vi "Stop Process.vi"(8 "error in (no error)":errorcluster, 11 "DLP2 in":refnum<class "DLP2.lvclass">) -> (0 "error out":errorcluster, 3 "DLP2 out":refnum<class "DLP2.lvclass">)   [LabVIEW 2022 SP3, in "DLP2.lvclass"]
doc: "Developed by Kevin Thompson\nkevin@thompsonengineering.net\n\nCopyright 2018\nThompson Engineering, LLC"
uses:
  DLP2.lvclass
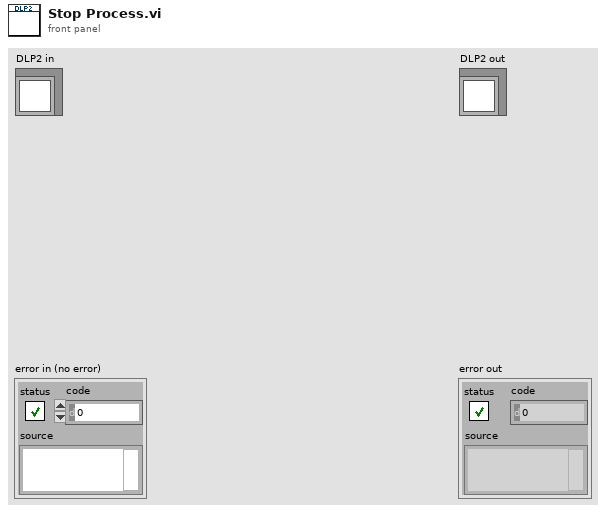
[diagram p1: front panel]
types:
  T1 = typedef "DLP2.lvclass/Public Events--cluster.ctl" = cluster{"Temp01.AsyncCmd Event":refnum<user-event>, "Temp01.AsyncMsg Event":refnum<user-event>, "stop process":refnum<user-event>, "API Incoming Event":refnum<user-event>, "API Executed Event":refnum<user-event>, "API Return Event":refnum<user-event>}
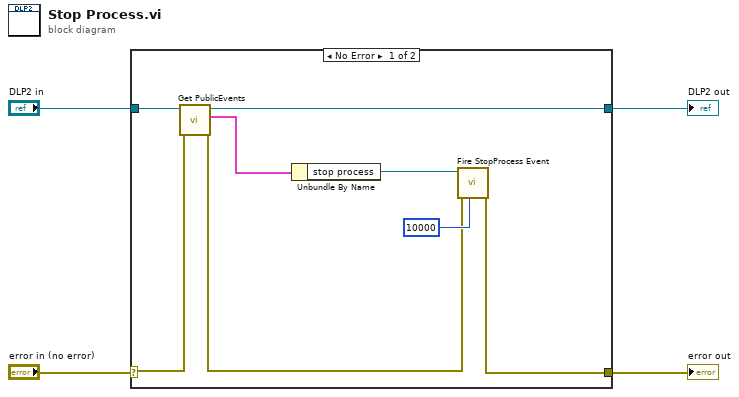
[diagram p0: block diagram]
diagram:
  n1 = case shown="No Error" "error in (no error)" {
    selector: "error in (no error)" -> [w6 w14]
    tunnel: [w12 w14] -> w3
    tunnel: [w11 w13] -> w1
    tunnel: "DLP2 in" -> [w10 w13]
    frame No Error {
      n2 = call "Get PublicEvents.vi"("error in (no error)"=w6, "DLP2 in"=w10) -> ("error out"=w5:errorcluster, "Public Events"=w9:T1, "DLP2 out"=w11:refnum<class "DLP2.lvclass">)  [unwired: 7 in]
      n3 = Unbundle By Name(w9) -> ("stop process"=w8:refnum<user-event>)
      n4 = call "Fire StopProcess Event.vi"("timeout in ms (5000)"=10000, "error in (no error)"=w5, "Event in"=w8) -> ("error out"=w12:errorcluster)  [unwired: 5 in, 3 out]
    }
    frame Error {
    }
  }
  "error out" <- w3
  "DLP2 out" <- w1
